vi "Live_Example_XCite.vi"() -> ()   [LabVIEW 2019]
doc: "An application to demonstrate the simultaneous control of a PCO camera and an X-Cite® light source\n\nUsage:\nSelect your required image count, data format and the camera setup before you start the program.\nOnce started, the camera class will be initialized and images will be recorded and displayed automatically\nYou can stop the images by pressing stop record.\nAfter stopped, the image at the selected index will be read out\nTo finish the program click on quit application, this will force an exit of the camera class\nYou can change your required ROI after and also during the record.\nA search for X-Cite® devices is started, and if found controls are initialized for each channel\nChannels can be switched on and off, and the intensity adjusted while the camera is acquiring images.\nWhen the recording is stopped, all the X-Cite® channels are switched off and controls are disabled.\n\n\nNote that this example will not be fail safe, i.e. doesnt react on errors, just handles them forward to the end"
uses:
  camera/Camera.lvclass
  pco.sdk/TimingControl/TimingControl.lvlib
  <vilib>/picture/picture.llb/Draw 8-Bit Pixmap.vi
  <vilib>/picture/picture.llb/Draw True-Color Pixmap.vi
  xcite/Xcite.lvclass
  <vilib>/Utility/miscctls.llb/LVOutOfRangeActionTypeDef.ctl
panel:
  in  "Channel9_On":bool caption="735 nm"
  in  "Channel9_Intensity":u32 caption="735 nm" min=5 max=100
  in  "Channel8_On":bool caption="635 nm"
  in  "Channel8_Intensity":u32 caption="635 nm" min=5 max=100
  in  "Channel7_On":bool caption="580 nm"
  in  "Channel7_Intensity":u32 caption="580 nm" min=5 max=100
  in  "Channel6_On":bool caption="555 nm"
  in  "Channel6_Intensity":u32 caption="555 nm" min=5 max=100
  in  "Channel5_On":bool caption="510 nm"
  in  "Channel5_Intensity":u32 caption="510 nm" min=5 max=100
  in  "Channel4_On":bool caption="550 nm"
  in  "Channel4_Intensity":u32 caption="550 nm" min=5 max=100
  in  "Channel3_On":bool caption="475 nm"
  in  "Channel3_Intensity":u32 caption="475 nm" min=5 max=100
  in  "Channel2_On":bool caption="430 nm"
  in  "Channel2_Intensity":u32 caption="430 nm" min=5 max=100
  in  "Channel1_On":bool caption="385 nm"
  in  "Channel1_Intensity":u32 caption="385 nm" min=5 max=100
  in  "type":u16(ring)=65535 items=["XC_120PC"=0, "XC_exacte"=1, "XC_120LED"=2, "XC_110LED"=3, "XC_mini"=4, "XC_XYLIS"=5, "XC_XR210"=6, "XC_LED1"=7, "XC_XT600"=8, "XC_XT900"=9, "Any"=65535]
  out "X-Cite® Model":u16(ring)=65535 items=["XC_120PC"=0, "XC_exacte"=1, "XC_120LED"=2, "XC_110LED"=3, "XC_mini"=4, "XC_XYLIS"=5, "XC_XR210"=6, "XC_LED1"=7, "XC_XT600"=8, "XC_XT900"=9, "Any"=65535]
  out "colormap(U8)":u32[](array[numeric])
  in  "Zoom [%]":i32(slide)=26 min=0 max=200 step=5 scale=10.0..200.0
  out "Image":picture
  out "Image(U16)":u16[][](graph)
  in  "Trigger":bool
  in  "data_format":T1(ring)=enum."Mono16"
  out "rawImage":u16[][](array[numeric])
  in  "Image Index":u32 max=9
  out "Recorded Images":u32
  in  "TriggerMode":T2(ring)
  in  "Quit":bool
  out "Error":errorcluster {"code" format="%x"}
  in  "Stop Record":bool
  out "Recording On":bool
  in  "cropY1":u64=2 min=1 max=2048 step=1
  in  "cropX1":u64=2 min=1 max=2048 step=1
  in  "cropY0":u64=1 min=1 max=2047 step=1
  in  "cropX0":u64=1 min=1 max=2047 step=1
  out "Image Height":u64
  out "Image Width":u64
  in  "dwImgCount":u32=10 caption="Required Number of Images" max=2397
  in  "Exposure Time [s]":dbl=0.010000000000000002 step=0.001
  # "This example demonstrates the image acquisition with one camera in ring buffer mode together with a live display of the latest images during record. Control of an X-Cite® light source is also possible. After recording is stopped, the images can be addressed by index.\nNote that this example will not be fail save, i.e. doesnt react on errors, just handles them forward to the end\n\nUsage:\nSelect your required image count, data format and the camera setup before you start the program.\nOnce started, the camera class will be initialized and images will be recorded and displayed automatically\nYou can stop the images by pressing stop record.\nAfter stopped, the image at the selected index will be read out\nTo finish the program click on quit application, this will force an exit of the camera class\nYou can change the cropped region during or after recording.\nA search for X-Cite® devices is started, and if found controls are initialized for each channel\nChannels can be switched on and off, and the intensity adjusted while the camera is acquiring images.\nWhen the recording is stopped, all the X-Cite® channels are switched off and controls are disabled."
  # "pco.labview"
  # "Camera Setup"
  # "X-Cite® controls"
  # "Recording Control"
  # "Parameters for image readout"
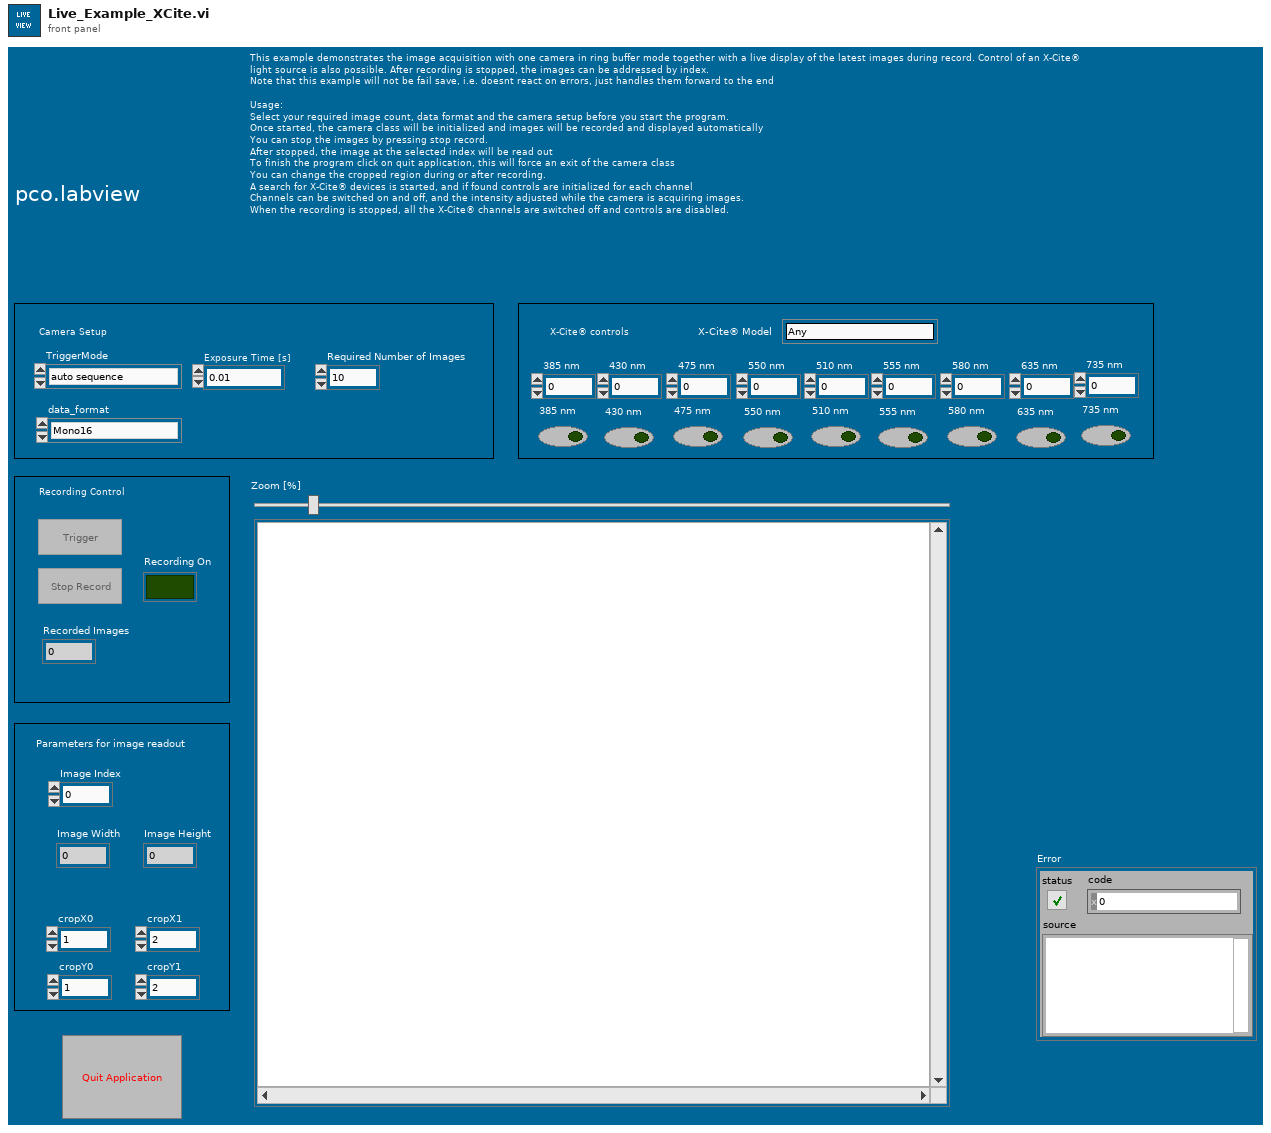
[diagram p1: front panel]
types:
  T1 = enum16{"Undefined", "Mono8", "Mono16", "BGRA8", "RGBA8", "BGRA16", "RGBA16", "CompressedMono8"}
  T2 = enum16{"auto sequence", "software trigger", "external exposure start", "external exposure control"}
  T3 = enum8{"Enabled", "Disabled", "Disabled and Grayed Out"}
  T4 = cluster{"serial":u32, "type":u16, "name":string, "wavelenghts_vec":u32[], "exclusivity_vec":u32[], "intensity_max_vec":u32[], "intensity_min_vec":u32[]}
  T5 = enum16{"sequence", "sequence non blocking", "ring buffer", "fifo", "tif", "multitif", "pcoraw", "b16", "dicom", "multidicom", "camram_ring", "camram_segment"}
  T6 = typedef "LVOutOfRangeActionTypeDef.ctl" = cluster{"Out of Range Action Minimum":u8, "Out of Range Action Maximum":u8, "Out of Range Action Increment":u8}
  T7 = cluster{"serial":u32, "type":u16, "sub_type":u16, "interface_type":u16, "bit_resolution":u16, "min_exposure_time_s":dbl, "max_exposure_time_s":dbl, "min_exposure_step_s":dbl, "min_delay_time_s":dbl, "max_delay_time_s":dbl, "min_delay_step_s":dbl, "min_width":u64, "min_height":u64, "max_width":u64, "max_height":u64, "roi_step_horz":u64, "roi_step_vert":u64, "roi_symmetric_horz":bool, "roi_symmetric_vert":bool, "has_timestamp_mode":bool, "has_timestamp_mode_ascii_only":bool, "pixelrate_vec":u32[], "conversion_factor_vec":sgl[], "has_trigger_mode_extexpctrl":bool, "has_acquire_mode":bool, "has_ext_acquire_mode":bool, "has_metadata_mode":bool, "has_ram":bool, "binning_horz_vec":u16[], "binning_vert_vec":u16[], "has_average_binning":bool, "pixel_format_vec":u32[]}
  T8 = cluster{"wSignalNum":u16, "wEnabled":u16, "wType":u16, "wPolarity":u16, "wFilterSetting":u16, "wSelected":u16, "dwParameter":u32[], "dwSignalFunctionality":u32[]}
  T9 = typedef "Camera.lvclass/binning.ctl" = cluster{"vert":u16, "horz":u16, "mode":u16}
  T10 = cluster{"exposure_time_s":dbl, "delay_time_s":dbl, "roi":cluster{"x0":u64, "y0":u64, "x1":u64, "y1":u64}, "timestamp_mode":u16, "pixelrate":u32, "conversion_factor":sgl, "trigger_mode":u16, "acquire_mode":u16, "acquire_sequence_number":u32, "metadata_mode":u16, "noisefilter_mode":u16, "pixel_format":u32, "binning":T9, "auto_exposure":cluster{"region":u16, "min_exposure_s":dbl, "max_exposure_s":dbl}}
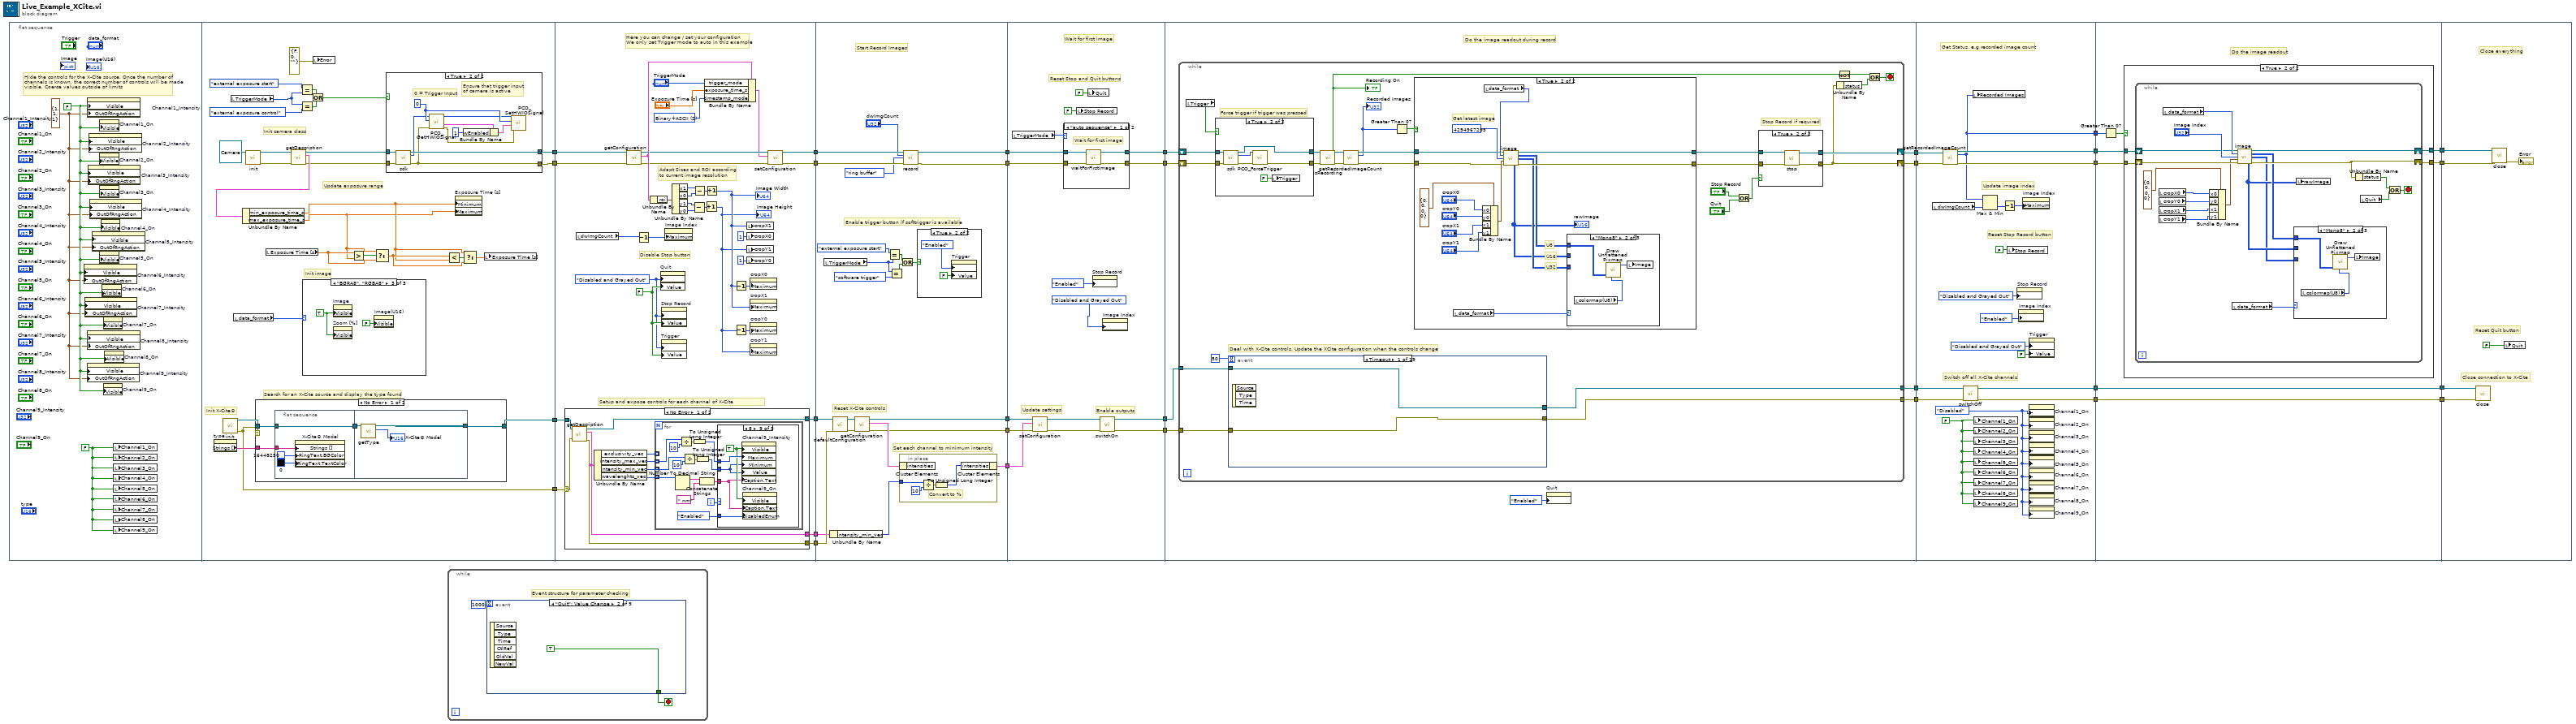
[diagram p0: block diagram]
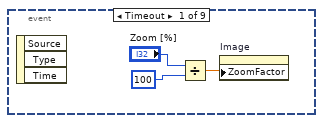
[diagram p2: hidden frame]
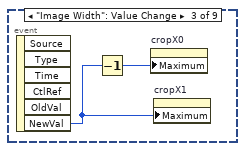
[diagram p3: hidden frame]
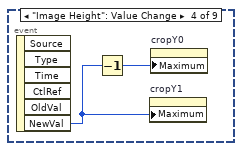
[diagram p4: hidden frame]
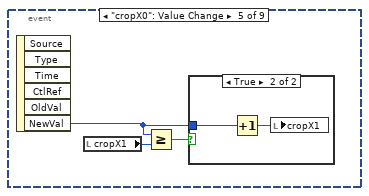
[diagram p5: hidden frame]
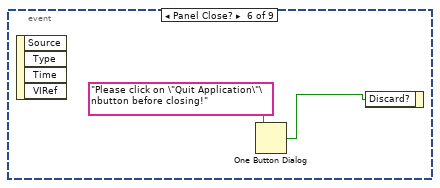
[diagram p7: hidden frame]
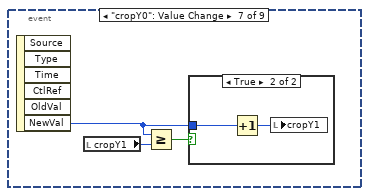
[diagram p8: hidden frame]
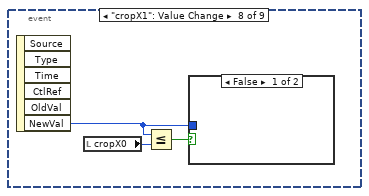
[diagram p10: hidden frame]
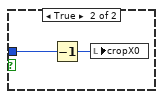
[diagram p11: hidden frame]
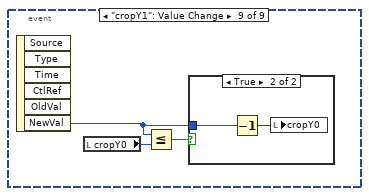
[diagram p12: hidden frame]
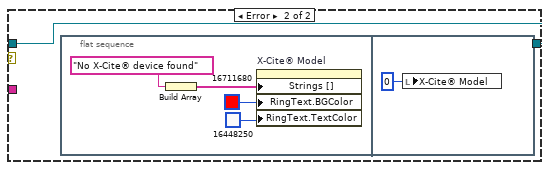
[diagram p14: hidden frame]
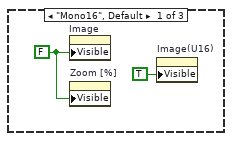
[diagram p16: hidden frame]
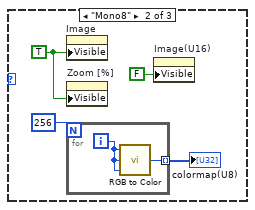
[diagram p17: hidden frame]
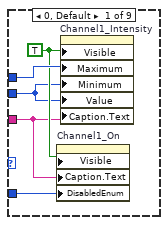
[diagram p18: hidden frame]
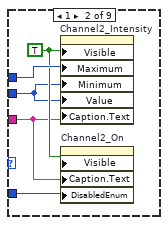
[diagram p19: hidden frame]
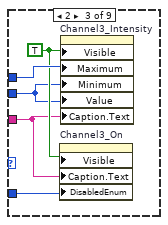
[diagram p20: hidden frame]
diagram:
  n1 = flat-sequence {
    tunnel: [w46] -> w23
    tunnel: [w39] -> w22
    tunnel: [w36] -> w16
    tunnel: [w35] -> w15
    tunnel: [w111] -> w31
    tunnel: [w115] -> w30
    tunnel: w23 -> [w110]
    tunnel: w22 -> [w109]
    tunnel: w16 -> [w105]
    tunnel: w15 -> [w106]
    tunnel: [w104] -> w14
    tunnel: [w103] -> w13
    tunnel: [w102] -> w9
    tunnel: [w217] -> w25
    tunnel: [w218] -> w24
    tunnel: w30 -> [w227]
    tunnel: w31 -> [w226]
    tunnel: w14 -> [w216]
    tunnel: w13 -> [w212]
    tunnel: w9 -> [w214]
    tunnel: [w210] -> w3
    tunnel: [w209] -> w2
    tunnel: [w207] -> w1
    tunnel: w25 -> [w245]
    tunnel: w24 -> [w246]
    tunnel: [w244] -> w29
    tunnel: [w242] -> w18
    tunnel: [w238] -> w12
    tunnel: [w239] -> w8
    tunnel: w3 -> [w236]
    tunnel: w2 -> [w240]
    tunnel: w1 -> [w234]
    tunnel: w29 -> [w264]
    tunnel: [w262] -> w28
    tunnel: [w261] -> w21
    tunnel: w18 -> [w260]
    tunnel: w12 -> [w259]
    tunnel: w8 -> [w258]
    tunnel: [w257] -> w7
    tunnel: [w256] -> w6
    tunnel: w28 -> [w609]
    tunnel: [w607] -> w27
    tunnel: w21 -> [w602]
    tunnel: [w601] -> w20
    tunnel: [w600] -> w17
    tunnel: [w599] -> w11
    tunnel: w7 -> [w598]
    tunnel: w6 -> [w597]
    tunnel: [w596] -> w5
    tunnel: w27 -> [w620]
    tunnel: [w619] -> w26
    tunnel: w20 -> [w618]
    tunnel: [w617] -> w19
    tunnel: w17 -> [w615]
    tunnel: w11 -> [w614]
    tunnel: [w614] -> w10
    tunnel: w5 -> [w613]
    tunnel: [w613] -> w4
    tunnel: w26 -> [w656]
    tunnel: w19 -> [w654]
    tunnel: w10 -> [w653]
    tunnel: w4 -> [w652]
    frame #0 {
      w32 = T6 {"Out of Range Action Minimum"=1, "Out of Range Action Maximum"=1, "Out of Range Action Increment"=1} ("Response to Value Outside Limits")
      w33 = FALSE
      w34 = FALSE
      # "Hide the controls for the X-Cite source. Once the number of channels is known, the correct number of controls will be made visible. Coerce values outside of limits"
      n2 = property on="Channel6_Intensity" class="DigNum (strict)"("Visible"=w34, "OutOfRngAction"=w32) -> ()  [unwired: 2 in, 2 out]
      n3 = property on="Channel7_Intensity" class="DigNum (strict)"("Visible"=w34, "OutOfRngAction"=w32) -> ()  [unwired: 2 in, 2 out]
      n4 = property on="Channel9_Intensity" class="DigNum (strict)"("Visible"=w34, "OutOfRngAction"=w32) -> ()  [unwired: 2 in, 2 out]
      n5 = property on="Channel1_Intensity" class="DigNum (strict)"("Visible"=w34, "OutOfRngAction"=w32) -> ()  [unwired: 2 in, 2 out]
      n6 = property on="Channel8_Intensity" class="DigNum (strict)"("Visible"=w34, "OutOfRngAction"=w32) -> ()  [unwired: 2 in, 2 out]
      n7 = property on="Channel3_Intensity" class="DigNum (strict)"("Visible"=w34, "OutOfRngAction"=w32) -> ()  [unwired: 2 in, 2 out]
      n8 = property on="Channel2_Intensity" class="DigNum (strict)"("Visible"=w34, "OutOfRngAction"=w32) -> ()  [unwired: 2 in, 2 out]
      n9 = property on="Channel4_Intensity" class="DigNum (strict)"("Visible"=w34, "OutOfRngAction"=w32) -> ()  [unwired: 2 in, 2 out]
      n10 = property on="Channel5_Intensity" class="DigNum (strict)"("Visible"=w34, "OutOfRngAction"=w32) -> ()  [unwired: 2 in, 2 out]
      n11 = property on="Channel2_On" class="Bool (strict)"("Visible"=w34) -> ()  [unwired: 2 in, 2 out]
      n12 = property on="Channel1_On" class="Bool (strict)"("Visible"=w34) -> ()  [unwired: 2 in, 2 out]
      n13 = property on="Channel3_On" class="Bool (strict)"("Visible"=w34) -> ()  [unwired: 2 in, 2 out]
      n14 = property on="Channel5_On" class="Bool (strict)"("Visible"=w34) -> ()  [unwired: 2 in, 2 out]
      n15 = property on="Channel4_On" class="Bool (strict)"("Visible"=w34) -> ()  [unwired: 2 in, 2 out]
      n16 = property on="Channel6_On" class="Bool (strict)"("Visible"=w34) -> ()  [unwired: 2 in, 2 out]
      n17 = property on="Channel7_On" class="Bool (strict)"("Visible"=w34) -> ()  [unwired: 2 in, 2 out]
      n18 = property on="Channel9_On" class="Bool (strict)"("Visible"=w34) -> ()  [unwired: 2 in, 2 out]
      n19 = property on="Channel8_On" class="Bool (strict)"("Visible"=w34) -> ()  [unwired: 2 in, 2 out]
      n20 = local write "Channel1_On"(w33) -> ()
      n21 = local write "Channel2_On"(w33) -> ()
      n22 = local write "Channel3_On"(w33) -> ()
      n23 = local write "Channel4_On"(w33) -> ()
      n24 = local write "Channel5_On"(w33) -> ()
      n25 = local write "Channel6_On"(w33) -> ()
      n26 = local write "Channel7_On"(w33) -> ()
      n27 = local write "Channel8_On"(w33) -> ()
      n28 = local write "Channel9_On"(w33) -> ()
    }
    frame #1 {
      # "Search for an X-Cite source and display the type found"
      # "Init X-Cite®"
      # "Init image"
      # "Init camera class"
      # "Update exposure range"
      n29 = property on="type" class="Ring (strict)"() -> ("Strings []"=w37:string[])  [unwired: 2 in, 2 out]
      n30 = call "init.vi"() -> ("error out"=w35:errorcluster, "Xcite out"=w38:refnum<class "Xcite.lvclass">)  [unwired: 10 in]
      n31 = local read "TriggerMode"() -> (w44:T2)
      n32 = local read "data_format"() -> (w49:T1)
      n33 = call-dynamic "init.vi"("Camera in"=refnum<class "Camera.lvclass"> refnum) -> ("Camera out"=w53:refnum<class "Camera.lvclass">, "error out"=w54:errorcluster)  [unwired: 8 in]
      n34 = case shown="No Error" w35 {
        tunnel: w38 -> [w63 w73]
        tunnel: [w64 w73] -> w36
        tunnel: w37 -> [w65 _]
        frame No Error {
          n35 = flat-sequence {
            tunnel: w65 -> [w69]
            tunnel: w63 -> [w68]
            tunnel: [w68] -> w62
            tunnel: [w72] -> w64
            tunnel: w62 -> [w70]
            frame #0 {
              n36 = property on="X-Cite® Model" class="Ring (strict)"("Strings []"=w69, "RingText.BGColor"=u32 16448250 ("Ring Text.Colors:BG Color"), "RingText.TextColor"=u32 0 ("Ring Text.Colors:FG Color")) -> ()  [unwired: 2 in, 2 out]
            }
            frame #1 {
              n37 = call "getType.vi"("Xcite in"=w70) -> ("type"=→"X-Cite® Model":u16, "Xcite out"=w72:refnum<class "Xcite.lvclass">)  [unwired: 8 in, 1 out]
            }
          }
        }
        frame Error {
          n38 = flat-sequence {
            frame #0 {
              n39 = Build Array("No X-Cite® device found") -> (w76:string[])
              n40 = property on="X-Cite® Model" class="Ring (strict)"("Strings []"=w76, "RingText.BGColor"=u32 16711680 ("Ring Text.Colors:BG Color"), "RingText.TextColor"=u32 16448250 ("Ring Text.Text Colors:Text Color")) -> ()  [unwired: 2 in, 2 out]
            }
            frame #1 {
              n41 = local write "X-Cite® Model"(0) -> ()
            }
          }
        }
      }
      n42 = local read "Exposure Time [s]"() -> (w60:dbl)
      n43 = call-dynamic "getDescription.vi"("error in (no error)"=w54, "Camera in"=w53) -> ("error out"=w48:errorcluster, "description"=w52:T7, "Camera out"=w47:refnum<class "Camera.lvclass">)  [unwired: 7 in]
      n44 = Unbundle By Name(w52) -> ("min_exposure_time_s"=w51:dbl, "max_exposure_time_s"=w50:dbl)
      n45 = Equal?(x=T2."external exposure start" ("TriggerMode"), y=w44) -> (x = y?=w42:bool)
      n46 = Equal?(x=w44, y=T2."external exposure control" ("TriggerMode")) -> (x = y?=w41:bool)
      n47 = case shown="\"BGRA8\", \"RGBA8\"" w49 {
        frame "Mono16", Default {
          w92 = FALSE ("Visible")
          n48 = property on="Image" class="Pict"("Visible"=w92) -> ()  [unwired: 2 in, 2 out]
          n49 = property on="Zoom [%]" class="Slide (strict)"("Visible"=w92) -> ()  [unwired: 2 in, 2 out]
          n50 = property on="Image(U16)" class="IntGraph (strict)"("Visible"=TRUE) -> ()  [unwired: 2 in, 2 out]
        }
        frame "Mono8" {
          w96 = TRUE ("Visible")
          n51 = property on="Image" class="Pict"("Visible"=w96) -> ()  [unwired: 2 in, 2 out]
          n52 = property on="Zoom [%]" class="Slide (strict)"("Visible"=w96) -> ()  [unwired: 2 in, 2 out]
          n53 = for {
            N: 256 -> [_]
            tunnel: [w98] -> w95 mode=indexing
            i -> [w99]
            n54 = call <vilib>:"RGB to Color.vi"("B"=w99, "G"=w99, "R"=w99) -> ("Color"=w98:u32)
          }
          "colormap(U8)" <- w95
          n55 = property on="Image(U16)" class="IntGraph (strict)"("Visible"=FALSE) -> ()  [unwired: 2 in, 2 out]
        }
        frame "BGRA8", "RGBA8" {
          w100 = TRUE ("Visible")
          n56 = property on="Image" class="Pict"("Visible"=w100) -> ()  [unwired: 2 in, 2 out]
          n57 = property on="Zoom [%]" class="Slide (strict)"("Visible"=w100) -> ()  [unwired: 2 in, 2 out]
          n58 = property on="Image(U16)" class="IntGraph (strict)"("Visible"=FALSE) -> ()  [unwired: 2 in, 2 out]
        }
      }
      n59 = Or(x=w42, y=w41) -> (x .or. y?=w40:bool)
      n60 = local write "Error"(errorcluster {"status"=FALSE, "code"=0, "source"=""} ("error IO")) -> ()
      n61 = Greater?(x=w60, y=w50) -> (0:w61:bool)
      n62 = Select(t=w50, s=w61, f=w60) -> (s? t:f=w58:dbl)
      n63 = case shown="True" w40 {
        tunnel: w48 -> [w79 w85]
        tunnel: w47 -> [w80 w84]
        tunnel: [w80 w83] -> w46
        tunnel: [w79 w81] -> w39
        frame False {
        }
        frame True {
          w89 = u16 0 ("wSignalNum")
          # "0 = Trigger Input"
          # "Ensure that trigger input\nof camera is active"
          n64 = call-dynamic "sdk.vi"("Camera in"=w84, "error in (no error)"=w85) -> ("Camera out"=w83:refnum<class "Camera.lvclass">, "sdk"=w82:u64, "error out"=w81:errorcluster)  [unwired: 11 in]
          n65 = call "PCO_GetHWIOSignal.vi"("error in (no error)"=w81, "wSignalNum"=w89, "ph"=w82) -> ("error out"=w87:errorcluster, "strSignal"=w91:T8, "ph out"=w86:u64)  [unwired: 5 in, 1 out]
          n66 = Bundle By Name(cluster=w91, "wEnabled"=u16 1) -> (w88:T8)
          n67 = call "PCO_SetHWIOSignal.vi"("error in (no error)"=w87, "strSignal"=w88, "wSignalNum"=w89, "ph"=w86) -> ()  [unwired: 5 in, 3 out]
        }
      }
      n68 = Less?(x=w58, y=w51) -> (x < y?=w59:bool)
      n69 = property on="Exposure Time [s]" class="DigNum (strict)"("Minimum"=w51, "Maximum"=w50) -> ()  [unwired: 2 in, 2 out]
      n70 = Select(t=w51, s=w59, f=w58) -> (s? t:f=w57:dbl)
      n71 = local write "Exposure Time [s]"(w57) -> ()
    }
    frame #2 {
      w121 = u16 2 items=["OFF", "Binary", "Binary+ASCII", "ASCII"] ("wTimeStampMode")
      w108 = FALSE ("Stop")
      w107 = T3."Disabled and Grayed Out" ("Disabled")
      # "Setup and expose controls for each channel of X-Cite"
      # "Disable Stop button"
      # "Adapt Sizes and ROI according\nto current image resolution"
      # "Here you can change / set your configuration\nWe only set Trigger mode to auto in this example"
      n72 = case shown="No Error" w106 {
        selector: w106 -> [w136 w203]
        tunnel: w105 -> [w143 w205]
        tunnel: [w142 w205] -> w104
        tunnel: [w137 T4 {"serial"=0, "type"=0, "name"="", "wavelenghts_vec"=[], "exclusivity_vec"=[], "intensity_max_vec"=[], "intensity_min_vec"=[]} ("XCITE_Description")] -> w103
        tunnel: [w135 w203] -> w102
        frame No Error {
          n73 = call "getDescription.vi"("error in (no error)"=w136, "Xcite in"=w143) -> ("error out"=w135:errorcluster, "description"=w137:T4, "Xcite out"=w142:refnum<class "Xcite.lvclass">)  [unwired: 7 in]
          n74 = Unbundle By Name(w137) -> ("exclusivity_vec"=w141:u32[], "intensity_max_vec"=w140:u32[], "intensity_min_vec"=w139:u32[], "wavelenghts_vec"=w138:u32[])
          n75 = for {
            tunnel: w141 -> [_] mode=indexing
            tunnel: w140 -> [w151] mode=indexing
            tunnel: w139 -> [w146] mode=indexing
            tunnel: w138 -> [w156] mode=indexing
            i -> [w157]
            n76 = Number To Decimal String(number=w156) -> (decimal integer string=w155:string)  [unwired: 1 in]
            n77 = Divide(x=w151, y=u32 10) -> (x/y=w149:dbl)
            n78 = Divide(x=w146, y=u32 10) -> (x/y=w147:dbl)
            n79 = To Unsigned Long Integer(number=w149) -> (unsigned 32bit integer=w144:u32)
            n80 = To Unsigned Long Integer(number=w147) -> (unsigned 32bit integer=w145:u32)
            n81 = Concatenate Strings(w155, " nm") -> (w153:string)
            n82 = case shown="8" w157 {
              tunnel: w153 -> [w159 w164 w169 w175 w180 w185 w189 w195 w200]
              tunnel: w144 -> [w162 w167 w172 w177 w182 w187 w192 w197 w202]
              tunnel: w145 -> [w160 w165 w170 w174 w179 w184 w190 w194 w199]
              tunnel: T3."Enabled" ("Disabled") -> [w158 w163 w168 w173 w178 w183 w188 w193 w198]
              frame 0, Default {
                w161 = TRUE ("Visible")
                n83 = property on="Channel1_On" class="Bool (strict)"("Visible"=w161, "Caption.Text"=w159, "DisabledEnum"=w158) -> ()  [unwired: 2 in, 2 out]
                n84 = property on="Channel1_Intensity" class="DigNum (strict)"("Visible"=w161, "Maximum"=w162, "Minimum"=w160, "Value"=w160, "Caption.Text"=w159) -> ()  [unwired: 2 in, 2 out]
              }
              frame 1 {
                w166 = TRUE ("Visible")
                n85 = property on="Channel2_Intensity" class="DigNum (strict)"("Visible"=w166, "Maximum"=w167, "Minimum"=w165, "Value"=w165, "Caption.Text"=w164) -> ()  [unwired: 2 in, 2 out]
                n86 = property on="Channel2_On" class="Bool (strict)"("Visible"=w166, "Caption.Text"=w164, "DisabledEnum"=w163) -> ()  [unwired: 2 in, 2 out]
              }
              frame 2 {
                w171 = TRUE ("Visible")
                n87 = property on="Channel3_On" class="Bool (strict)"("Visible"=w171, "Caption.Text"=w169, "DisabledEnum"=w168) -> ()  [unwired: 2 in, 2 out]
                n88 = property on="Channel3_Intensity" class="DigNum (strict)"("Visible"=w171, "Maximum"=w172, "Minimum"=w170, "Value"=w170, "Caption.Text"=w169) -> ()  [unwired: 2 in, 2 out]
              }
              frame 3 {
                w176 = TRUE ("Visible")
                n89 = property on="Channel4_Intensity" class="DigNum (strict)"("Visible"=w176, "Maximum"=w177, "Minimum"=w174, "Value"=w174, "Caption.Text"=w175) -> ()  [unwired: 2 in, 2 out]
                n90 = property on="Channel4_On" class="Bool (strict)"("Visible"=w176, "Caption.Text"=w175, "DisabledEnum"=w173) -> ()  [unwired: 2 in, 2 out]
              }
              frame 4 {
                w181 = TRUE ("Visible")
                n91 = property on="Channel5_Intensity" class="DigNum (strict)"("Visible"=w181, "Maximum"=w182, "Minimum"=w179, "Value"=w179, "Caption.Text"=w180) -> ()  [unwired: 2 in, 2 out]
                n92 = property on="Channel5_On" class="Bool (strict)"("Visible"=w181, "Caption.Text"=w180, "DisabledEnum"=w178) -> ()  [unwired: 2 in, 2 out]
              }
              frame 5 {
                w186 = TRUE ("Visible")
                n93 = property on="Channel6_Intensity" class="DigNum (strict)"("Visible"=w186, "Maximum"=w187, "Minimum"=w184, "Value"=w184, "Caption.Text"=w185) -> ()  [unwired: 2 in, 2 out]
                n94 = property on="Channel6_On" class="Bool (strict)"("Visible"=w186, "Caption.Text"=w185, "DisabledEnum"=w183) -> ()  [unwired: 2 in, 2 out]
              }
              frame 6 {
                w191 = TRUE ("Visible")
                n95 = property on="Channel7_Intensity" class="DigNum (strict)"("Visible"=w191, "Maximum"=w192, "Minimum"=w190, "Value"=w190, "Caption.Text"=w189) -> ()  [unwired: 2 in, 2 out]
                n96 = property on="Channel7_On" class="Bool (strict)"("Visible"=w191, "Caption.Text"=w189, "DisabledEnum"=w188) -> ()  [unwired: 2 in, 2 out]
              }
              frame 7 {
                w196 = TRUE ("Visible")
                n97 = property on="Channel8_Intensity" class="DigNum (strict)"("Visible"=w196, "Maximum"=w197, "Minimum"=w194, "Value"=w194, "Caption.Text"=w195) -> ()  [unwired: 2 in, 2 out]
                n98 = property on="Channel8_On" class="Bool (strict)"("Visible"=w196, "Caption.Text"=w195, "DisabledEnum"=w193) -> ()  [unwired: 2 in, 2 out]
              }
              frame 8 {
                w201 = TRUE ("Visible")
                n99 = property on="Channel9_Intensity" class="DigNum (strict)"("Visible"=w201, "Maximum"=w202, "Minimum"=w199, "Value"=w199, "Caption.Text"=w200) -> ()  [unwired: 2 in, 2 out]
                n100 = property on="Channel9_On" class="Bool (strict)"("Visible"=w201, "Caption.Text"=w200, "DisabledEnum"=w198) -> ()  [unwired: 2 in, 2 out]
              }
            }
          }
        }
        frame Error {
        }
      }
      n101 = local read "dwImgCount"() -> (w122:u32)
      n102 = call-dynamic "getConfiguration.vi"("error in (no error)"=w109, "Camera in"=w110) -> ("error out"=w116:errorcluster, "configuration"=w127:T10, "Camera out"=w118:refnum<class "Camera.lvclass">)  [unwired: 7 in]
      n103 = Decrement(x=w122) -> (x-1=w112:u32)
      n104 = Unbundle By Name(w127) -> ("roi"=w128:cluster{"x0":u64, "y0":u64, "x1":u64, "y1":u64})
      n105 = property on="Quit" class="Bool (strict)"("DisabledEnum"=w107, "Value"=w108) -> ()  [unwired: 2 in, 2 out]
      n106 = property on="Stop Record" class="Bool (strict)"("DisabledEnum"=w107, "Value"=w108) -> ()  [unwired: 2 in, 2 out]
      n107 = property on="Trigger" class="Bool (strict)"("DisabledEnum"=w107, "Value"=w108) -> ()  [unwired: 2 in, 2 out]
      n108 = property on="Image Index" class="DigNum (strict)"("Maximum"=w112) -> ()  [unwired: 2 in, 2 out]
      n109 = Unbundle By Name(w128) -> ("x1"=w130:u64, "x0"=w129:u64, "y1"=w132:u64, "y0"=w131:u64)
      n110 = Subtract(x=w132, y=w131) -> (x-y=w134:u64)
      n111 = Subtract(x=w130, y=w129) -> (x-y=w133:u64)
      n112 = Bundle By Name(cluster=w127, "trigger_mode"="TriggerMode", "exposure_time_s"="Exposure Time [s]", "timestamp_mode"=w121) -> (w117:T10)
      n113 = Increment(x=w134) -> (x+1=w113:u64)
      "Image Height" <- w113
      n114 = Increment(x=w133) -> (x+1=w114:u64)
      "Image Width" <- w114
      n115 = Decrement(x=w114) -> (x-1=w125:u64)
      n116 = Decrement(x=w113) -> (x-1=w126:u64)
      n117 = local write "cropX1"(w114) -> ()
      n118 = local write "cropX0"(u64 1 ("roiY0")) -> ()
      n119 = local write "cropY1"(w113) -> ()
      n120 = local write "cropY0"(u64 1 ("roiY0")) -> ()
      n121 = property on="cropX0" class="DigNum (strict)"("Maximum"=w125) -> ()  [unwired: 2 in, 2 out]
      n122 = property on="cropX1" class="DigNum (strict)"("Maximum"=w114) -> ()  [unwired: 2 in, 2 out]
      n123 = property on="cropY0" class="DigNum (strict)"("Maximum"=w126) -> ()  [unwired: 2 in, 2 out]
      n124 = property on="cropY1" class="DigNum (strict)"("Maximum"=w113) -> ()  [unwired: 2 in, 2 out]
      n125 = call-dynamic "setConfiguration.vi"("error in (no error)"=w116, "configuration"=w117, "Camera in"=w118) -> ("error out"=w115:errorcluster, "Camera out"=w111:refnum<class "Camera.lvclass">)  [unwired: 7 in]
    }
    frame #3 {
      # "Set each channel to minimum intensity"
      # "Reset X-Cite controls"
      # "Enable trigger button if softtrigger is available"
      # "Start Record Images"
      n126 = local read "TriggerMode"() -> (w223:T2)
      n127 = Unbundle By Name(w212) -> ("intensity_min_vec"=w208:u32[])
      n128 = call "defaultConfiguration.vi"("error in (no error)"=w214, "Xcite in"=w216) -> ("error out"=w213:errorcluster, "Xcite out"=w215:refnum<class "Xcite.lvclass">)  [unwired: 8 in]
      n129 = call "getConfiguration.vi"("error in (no error)"=w213, "Xcite in"=w215) -> ("error out"=w210:errorcluster, "configuration"=w211:cluster{"intensities":u32[], "on_states":u8[]}, "Xcite out"=w209:refnum<class "Xcite.lvclass">)  [unwired: 7 in]
      n130 = Equal?(x=T2."external exposure start" ("TriggerMode"), y=w223) -> (x = y?=w220:bool)
      n131 = Equal?(x=w223, y=T2."software trigger" ("TriggerMode")) -> (x = y?=w219:bool)
      n132 = in-place {
        in-place-border: w208 -> [w229]
        # "Convert to %"
        n133 = in-place-cluster #1(w211) -> ()  [unwired: 1 out]
        n134 = Divide(x=w229, y=u32 10) -> (x/y=w230:dbl[])
        n135 = To Unsigned Long Integer(number=w230) -> (unsigned 32bit integer=w228:u32[])
        n136 = in-place-cluster #1("intensities"=w228) -> (w207:cluster{"intensities":u32[], "on_states":u8[]})
      }
      n137 = Or(x=w220, y=w219) -> (x .or. y?=w221:bool)
      n138 = call-dynamic "record.vi"("Camera in"=w226, "num_images"="dwImgCount", "record_mode"=T5."ring buffer", "error in (no error)"=w227) -> ("Camera out"=w218:refnum<class "Camera.lvclass">, "error out"=w217:errorcluster)  [unwired: 10 in]
      n139 = case shown="True" w221 {
        frame False {
        }
        frame True {
          n140 = property on="Trigger" class="Bool (strict)"("DisabledEnum"=T3."Enabled" ("Disabled"), "Value"=FALSE ("Trigger")) -> ()  [unwired: 2 in, 2 out]
        }
      }
    }
    frame #4 {
      # "Enable outputs"
      # "Update settings"
      # "Wait for first image"
      # "Reset Stop and Quit buttons"
      n141 = local read "TriggerMode"() -> (w241:T2)
      n142 = call "setConfiguration.vi"("error in (no error)"=w236, "configuration"=w234, "Xcite in"=w240) -> ("error out"=w235:errorcluster, "Xcite out"=w237:refnum<class "Xcite.lvclass">)  [unwired: 7 in]
      n143 = case shown="\"auto sequence\"" w241 {
        tunnel: w246 -> [w253 w255]
        tunnel: w245 -> [w252 w254]
        tunnel: [w251 w254] -> w244
        tunnel: [w250 w255] -> w242
        frame "auto sequence" {
          # "Wait for first image"
          n144 = call-dynamic "waitForFirstImage.vi"("error in (no error)"=w252, "Camera in"=w253) -> ("error out"=w251:errorcluster, "Camera out"=w250:refnum<class "Camera.lvclass">)  [unwired: 8 in]
        }
        frame Default {
        }
      }
      n145 = local write "Stop Record"(FALSE ("Stop Record")) -> ()
      n146 = local write "Quit"(FALSE ("Stop")) -> ()
      n147 = property on="Stop Record" class="Bool (strict)"("DisabledEnum"=T3."Enabled" ("Disabled")) -> ()  [unwired: 2 in, 2 out]
      n148 = call "switchOn.vi"("error in (no error)"=w235, "Xcite in"=w237) -> ("error out"=w239:errorcluster, "Xcite out"=w238:refnum<class "Xcite.lvclass">)  [unwired: 8 in]
      n149 = property on="Image Index" class="DigNum (strict)"("DisabledEnum"=T3."Disabled and Grayed Out" ("Disabled")) -> ()  [unwired: 2 in, 2 out]
    }
    frame #5 {
      # "Do the image readout during record"
      n150 = while {
        shift-right: [w272] -> w262
        shift-left: w264 -> [w276]
        shift-right: [w273] -> w261
        shift-left: w260 -> [w277]
        tunnel: w259 -> [w268]
        tunnel: w258 -> [w267]
        tunnel: [w266] -> w257
        tunnel: [w265] -> w256
        stop <- w288 stop-if-true
        # "Deal with X-Cite controls. Update the XCite configuration when the controls change"
        # "Force trigger if trigger was pressed"
        # "Stop Record if required"
        n151 = local read "Trigger"() -> (w278:bool)
        n152 = case shown="True" w278 {
          tunnel: w277 -> [w580 w585]
          tunnel: w276 -> [w579 w584]
          tunnel: [w580 w583] -> w275
          tunnel: [w579 w582] -> w274
          frame False {
          }
          frame True {
            n153 = call-dynamic "sdk.vi"("Camera in"=w585, "error in (no error)"=w584) -> ("Camera out"=w583:refnum<class "Camera.lvclass">, "sdk"=w586:u64, "error out"=w587:errorcluster)  [unwired: 11 in]
            n154 = call "PCO_ForceTrigger.vi"("error in (no error)"=w587, "ph"=w586) -> ("error out"=w582:errorcluster)  [unwired: 6 in, 3 out]
            n155 = local write "Trigger"(FALSE ("Trigger")) -> ()
          }
        }
        n156 = event shown="[0] Timeout" {
          selector: _ -> [_ _ _ _ _ _ _ _ _ _ _ _ _ _ _ _ _ _ _]
          dyn-events: _ -> [_ _ _ _ _ _ _ _ _ _ _ _ _ _ _ _ _ _ _]
          timeout: 50 -> [_ _ _ _ _ _ _ _ _ _ _ _ _ _ _ _ _ _ _]
          tunnel: w268 -> [w292 w300 w315 w330 w345 w360 w375 w390 w405 w420 w436 w450 w464 w478 w492 w506 w520 w534 w548]
          tunnel: [w293 w299 w314 w329 w344 w359 w374 w389 w404 w419 w435 w449 w463 w477 w491 w505 w519 w533 w547] -> w265
          tunnel: w267 -> [w293 w295 w310 w325 w340 w355 w370 w385 w400 w415 w430 w444 w458 w472 w486 w500 w514 w528 w542]
          tunnel: [w292 w298 w313 w328 w343 w358 w373 w388 w403 w418 w434 w448 w462 w476 w490 w504 w518 w532 w546] -> w266
          event Timeout {
            n157 = event-data() -> ()  [unwired: 1 in, 3 out]
          }
          event "Channel1_Intensity": Value Change {
            n158 = event-data() -> ("NewVal"=w302:u32)  [unwired: 1 in, 5 out]
            n159 = call "getConfiguration.vi"("error in (no error)"=w295, "Xcite in"=w300) -> ("error out"=w294:errorcluster, "configuration"=w296:cluster{"intensities":u32[], "on_states":u8[]}, "Xcite out"=w297:refnum<class "Xcite.lvclass">)  [unwired: 7 in]
            n160 = in-place {
              in-place-border: w302 -> [w306]
              # "Convert to permille"
              n161 = in-place-cluster #2(w296) -> ("intensities"=w308:u32[])
              n162 = Replace Array Subset(array=w308, new element=w306, index=0) -> (w304:u32[])
              n163 = Multiply(x=w304, y=u32 10) -> (x*y=w303:u32[])
              n164 = in-place-cluster #2("intensities"=w303) -> (w301:cluster{"intensities":u32[], "on_states":u8[]})
            }
            n165 = call "setConfiguration.vi"("error in (no error)"=w294, "configuration"=w301, "Xcite in"=w297) -> ("error out"=w299:errorcluster, "Xcite out"=w298:refnum<class "Xcite.lvclass">)  [unwired: 7 in]
          }
          event "Channel2_Intensity": Value Change {
            n166 = event-data() -> ("NewVal"=w317:u32)  [unwired: 1 in, 5 out]
            n167 = call "getConfiguration.vi"("error in (no error)"=w310, "Xcite in"=w315) -> ("error out"=w309:errorcluster, "configuration"=w311:cluster{"intensities":u32[], "on_states":u8[]}, "Xcite out"=w312:refnum<class "Xcite.lvclass">)  [unwired: 7 in]
            n168 = in-place {
              in-place-border: w317 -> [w321]
              # "Convert to permille"
              n169 = in-place-cluster #3(w311) -> ("intensities"=w323:u32[])
              n170 = Replace Array Subset(array=w323, new element=w321, index=1) -> (w319:u32[])
              n171 = Multiply(x=w319, y=u32 10) -> (x*y=w318:u32[])
              n172 = in-place-cluster #3("intensities"=w318) -> (w316:cluster{"intensities":u32[], "on_states":u8[]})
            }
            n173 = call "setConfiguration.vi"("error in (no error)"=w309, "configuration"=w316, "Xcite in"=w312) -> ("error out"=w314:errorcluster, "Xcite out"=w313:refnum<class "Xcite.lvclass">)  [unwired: 7 in]
          }
          event "Channel3_Intensity": Value Change {
            n174 = event-data() -> ("NewVal"=w332:u32)  [unwired: 1 in, 5 out]
            n175 = call "getConfiguration.vi"("error in (no error)"=w325, "Xcite in"=w330) -> ("error out"=w324:errorcluster, "configuration"=w326:cluster{"intensities":u32[], "on_states":u8[]}, "Xcite out"=w327:refnum<class "Xcite.lvclass">)  [unwired: 7 in]
            n176 = in-place {
              in-place-border: w332 -> [w336]
              # "Convert to permille"
              n177 = in-place-cluster #4(w326) -> ("intensities"=w338:u32[])
              n178 = Replace Array Subset(array=w338, new element=w336, index=2) -> (w334:u32[])
              n179 = Multiply(x=w334, y=u32 10) -> (x*y=w333:u32[])
              n180 = in-place-cluster #4("intensities"=w333) -> (w331:cluster{"intensities":u32[], "on_states":u8[]})
            }
            n181 = call "setConfiguration.vi"("error in (no error)"=w324, "configuration"=w331, "Xcite in"=w327) -> ("error out"=w329:errorcluster, "Xcite out"=w328:refnum<class "Xcite.lvclass">)  [unwired: 7 in]
          }
          event "Channel4_Intensity": Value Change {
            n182 = event-data() -> ("NewVal"=w347:u32)  [unwired: 1 in, 5 out]
            n183 = call "getConfiguration.vi"("error in (no error)"=w340, "Xcite in"=w345) -> ("error out"=w339:errorcluster, "configuration"=w341:cluster{"intensities":u32[], "on_states":u8[]}, "Xcite out"=w342:refnum<class "Xcite.lvclass">)  [unwired: 7 in]
            n184 = in-place {
              in-place-border: w347 -> [w351]
              # "Convert to permille"
              n185 = in-place-cluster #5(w341) -> ("intensities"=w353:u32[])
              n186 = Replace Array Subset(array=w353, new element=w351, index=3) -> (w349:u32[])
              n187 = Multiply(x=w349, y=u32 10) -> (x*y=w348:u32[])
              n188 = in-place-cluster #5("intensities"=w348) -> (w346:cluster{"intensities":u32[], "on_states":u8[]})
            }
            n189 = call "setConfiguration.vi"("error in (no error)"=w339, "configuration"=w346, "Xcite in"=w342) -> ("error out"=w344:errorcluster, "Xcite out"=w343:refnum<class "Xcite.lvclass">)  [unwired: 7 in]
          }
          event "Channel5_Intensity": Value Change {
            n190 = event-data() -> ("NewVal"=w362:u32)  [unwired: 1 in, 5 out]
            n191 = call "getConfiguration.vi"("error in (no error)"=w355, "Xcite in"=w360) -> ("error out"=w354:errorcluster, "configuration"=w356:cluster{"intensities":u32[], "on_states":u8[]}, "Xcite out"=w357:refnum<class "Xcite.lvclass">)  [unwired: 7 in]
            n192 = in-place {
              in-place-border: w362 -> [w366]
              # "Convert to permille"
              n193 = in-place-cluster #6(w356) -> ("intensities"=w368:u32[])
              n194 = Replace Array Subset(array=w368, new element=w366, index=4) -> (w364:u32[])
              n195 = Multiply(x=w364, y=u32 10) -> (x*y=w363:u32[])
              n196 = in-place-cluster #6("intensities"=w363) -> (w361:cluster{"intensities":u32[], "on_states":u8[]})
            }
            n197 = call "setConfiguration.vi"("error in (no error)"=w354, "configuration"=w361, "Xcite in"=w357) -> ("error out"=w359:errorcluster, "Xcite out"=w358:refnum<class "Xcite.lvclass">)  [unwired: 7 in]
          }
          event "Channel6_Intensity": Value Change {
            n198 = event-data() -> ("NewVal"=w377:u32)  [unwired: 1 in, 5 out]
            n199 = call "getConfiguration.vi"("error in (no error)"=w370, "Xcite in"=w375) -> ("error out"=w369:errorcluster, "configuration"=w371:cluster{"intensities":u32[], "on_states":u8[]}, "Xcite out"=w372:refnum<class "Xcite.lvclass">)  [unwired: 7 in]
            n200 = in-place {
              in-place-border: w377 -> [w381]
              # "Convert to permille"
              n201 = in-place-cluster #7(w371) -> ("intensities"=w383:u32[])
              n202 = Replace Array Subset(array=w383, new element=w381, index=5) -> (w379:u32[])
              n203 = Multiply(x=w379, y=u32 10) -> (x*y=w378:u32[])
              n204 = in-place-cluster #7("intensities"=w378) -> (w376:cluster{"intensities":u32[], "on_states":u8[]})
            }
            n205 = call "setConfiguration.vi"("error in (no error)"=w369, "configuration"=w376, "Xcite in"=w372) -> ("error out"=w374:errorcluster, "Xcite out"=w373:refnum<class "Xcite.lvclass">)  [unwired: 7 in]
          }
          event "Channel7_Intensity": Value Change {
            n206 = event-data() -> ("NewVal"=w392:u32)  [unwired: 1 in, 5 out]
            n207 = call "getConfiguration.vi"("error in (no error)"=w385, "Xcite in"=w390) -> ("error out"=w384:errorcluster, "configuration"=w386:cluster{"intensities":u32[], "on_states":u8[]}, "Xcite out"=w387:refnum<class "Xcite.lvclass">)  [unwired: 7 in]
            n208 = in-place {
              in-place-border: w392 -> [w396]
              # "Convert to permille"
              n209 = in-place-cluster #8(w386) -> ("intensities"=w398:u32[])
              n210 = Replace Array Subset(array=w398, new element=w396, index=6) -> (w394:u32[])
              n211 = Multiply(x=w394, y=u32 10) -> (x*y=w393:u32[])
              n212 = in-place-cluster #8("intensities"=w393) -> (w391:cluster{"intensities":u32[], "on_states":u8[]})
            }
            n213 = call "setConfiguration.vi"("error in (no error)"=w384, "configuration"=w391, "Xcite in"=w387) -> ("error out"=w389:errorcluster, "Xcite out"=w388:refnum<class "Xcite.lvclass">)  [unwired: 7 in]
          }
          event "Channel8_Intensity": Value Change {
            n214 = event-data() -> ("NewVal"=w407:u32)  [unwired: 1 in, 5 out]
            n215 = call "getConfiguration.vi"("error in (no error)"=w400, "Xcite in"=w405) -> ("error out"=w399:errorcluster, "configuration"=w401:cluster{"intensities":u32[], "on_states":u8[]}, "Xcite out"=w402:refnum<class "Xcite.lvclass">)  [unwired: 7 in]
            n216 = in-place {
              in-place-border: w407 -> [w411]
              # "Convert to permille"
              n217 = in-place-cluster #9(w401) -> ("intensities"=w413:u32[])
              n218 = Replace Array Subset(array=w413, new element=w411, index=7) -> (w409:u32[])
              n219 = Multiply(x=w409, y=u32 10) -> (x*y=w408:u32[])
              n220 = in-place-cluster #9("intensities"=w408) -> (w406:cluster{"intensities":u32[], "on_states":u8[]})
            }
            n221 = call "setConfiguration.vi"("error in (no error)"=w399, "configuration"=w406, "Xcite in"=w402) -> ("error out"=w404:errorcluster, "Xcite out"=w403:refnum<class "Xcite.lvclass">)  [unwired: 7 in]
          }
          event "Channel9_Intensity": Value Change {
            n222 = event-data() -> ("NewVal"=w422:u32)  [unwired: 1 in, 5 out]
            n223 = call "getConfiguration.vi"("error in (no error)"=w415, "Xcite in"=w420) -> ("error out"=w414:errorcluster, "configuration"=w416:cluster{"intensities":u32[], "on_states":u8[]}, "Xcite out"=w417:refnum<class "Xcite.lvclass">)  [unwired: 7 in]
            n224 = in-place {
              in-place-border: w422 -> [w426]
              # "Convert to permille"
              n225 = in-place-cluster #10(w416) -> ("intensities"=w428:u32[])
              n226 = Replace Array Subset(array=w428, new element=w426, index=8) -> (w424:u32[])
              n227 = Multiply(x=w424, y=u32 10) -> (x*y=w423:u32[])
              n228 = in-place-cluster #10("intensities"=w423) -> (w421:cluster{"intensities":u32[], "on_states":u8[]})
            }
            n229 = call "setConfiguration.vi"("error in (no error)"=w414, "configuration"=w421, "Xcite in"=w417) -> ("error out"=w419:errorcluster, "Xcite out"=w418:refnum<class "Xcite.lvclass">)  [unwired: 7 in]
          }
          event "Channel1_On": Value Change {
            n230 = event-data() -> ("NewVal"=w438:bool)  [unwired: 1 in, 5 out]
            n231 = call "getConfiguration.vi"("error in (no error)"=w430, "Xcite in"=w436) -> ("error out"=w429:errorcluster, "configuration"=w432:cluster{"intensities":u32[], "on_states":u8[]}, "Xcite out"=w433:refnum<class "Xcite.lvclass">)  [unwired: 7 in]
            n232 = Boolean To (0,1)(Boolean=w438) -> (0, 1=w431:i16)
            n233 = in-place {
              in-place-border: w431 -> [w439]
              n234 = in-place-cluster #11(w432) -> ("on_states"=w442:u8[])
              n235 = Replace Array Subset(array=w442, new element=w439, index=0) -> (w441:u8[])
              n236 = in-place-cluster #11("on_states"=w441) -> (w437:cluster{"intensities":u32[], "on_states":u8[]})
            }
            n237 = call "setConfiguration.vi"("error in (no error)"=w429, "configuration"=w437, "Xcite in"=w433) -> ("error out"=w435:errorcluster, "Xcite out"=w434:refnum<class "Xcite.lvclass">)  [unwired: 7 in]
          }
          event "Channel2_On": Value Change {
            n238 = event-data() -> ("NewVal"=w452:bool)  [unwired: 1 in, 5 out]
            n239 = Boolean To (0,1)(Boolean=w452) -> (0, 1=w445:i16)
            n240 = call "getConfiguration.vi"("error in (no error)"=w444, "Xcite in"=w450) -> ("error out"=w443:errorcluster, "configuration"=w446:cluster{"intensities":u32[], "on_states":u8[]}, "Xcite out"=w447:refnum<class "Xcite.lvclass">)  [unwired: 7 in]
            n241 = in-place {
              in-place-border: w445 -> [w453]
              n242 = in-place-cluster #12(w446) -> ("on_states"=w456:u8[])
              n243 = Replace Array Subset(array=w456, new element=w453, index=1) -> (w455:u8[])
              n244 = in-place-cluster #12("on_states"=w455) -> (w451:cluster{"intensities":u32[], "on_states":u8[]})
            }
            n245 = call "setConfiguration.vi"("error in (no error)"=w443, "configuration"=w451, "Xcite in"=w447) -> ("error out"=w449:errorcluster, "Xcite out"=w448:refnum<class "Xcite.lvclass">)  [unwired: 7 in]
          }
          event "Channel3_On": Value Change {
            n246 = event-data() -> ("NewVal"=w466:bool)  [unwired: 1 in, 5 out]
            n247 = call "getConfiguration.vi"("error in (no error)"=w458, "Xcite in"=w464) -> ("error out"=w457:errorcluster, "configuration"=w460:cluster{"intensities":u32[], "on_states":u8[]}, "Xcite out"=w461:refnum<class "Xcite.lvclass">)  [unwired: 7 in]
            n248 = Boolean To (0,1)(Boolean=w466) -> (0, 1=w459:i16)
            n249 = in-place {
              in-place-border: w459 -> [w467]
              n250 = in-place-cluster #13(w460) -> ("on_states"=w470:u8[])
              n251 = Replace Array Subset(array=w470, new element=w467, index=2) -> (w469:u8[])
              n252 = in-place-cluster #13("on_states"=w469) -> (w465:cluster{"intensities":u32[], "on_states":u8[]})
            }
            n253 = call "setConfiguration.vi"("error in (no error)"=w457, "configuration"=w465, "Xcite in"=w461) -> ("error out"=w463:errorcluster, "Xcite out"=w462:refnum<class "Xcite.lvclass">)  [unwired: 7 in]
          }
          event "Channel4_On": Value Change {
            n254 = event-data() -> ("NewVal"=w480:bool)  [unwired: 1 in, 5 out]
            n255 = call "getConfiguration.vi"("error in (no error)"=w472, "Xcite in"=w478) -> ("error out"=w471:errorcluster, "configuration"=w474:cluster{"intensities":u32[], "on_states":u8[]}, "Xcite out"=w475:refnum<class "Xcite.lvclass">)  [unwired: 7 in]
            n256 = Boolean To (0,1)(Boolean=w480) -> (0, 1=w473:i16)
            n257 = in-place {
              in-place-border: w473 -> [w481]
              n258 = in-place-cluster #14(w474) -> ("on_states"=w484:u8[])
              n259 = Replace Array Subset(array=w484, new element=w481, index=3) -> (w483:u8[])
              n260 = in-place-cluster #14("on_states"=w483) -> (w479:cluster{"intensities":u32[], "on_states":u8[]})
            }
            n261 = call "setConfiguration.vi"("error in (no error)"=w471, "configuration"=w479, "Xcite in"=w475) -> ("error out"=w477:errorcluster, "Xcite out"=w476:refnum<class "Xcite.lvclass">)  [unwired: 7 in]
          }
          event "Channel5_On": Value Change {
            n262 = event-data() -> ("NewVal"=w494:bool)  [unwired: 1 in, 5 out]
            n263 = call "getConfiguration.vi"("error in (no error)"=w486, "Xcite in"=w492) -> ("error out"=w485:errorcluster, "configuration"=w488:cluster{"intensities":u32[], "on_states":u8[]}, "Xcite out"=w489:refnum<class "Xcite.lvclass">)  [unwired: 7 in]
            n264 = Boolean To (0,1)(Boolean=w494) -> (0, 1=w487:i16)
            n265 = in-place {
              in-place-border: w487 -> [w495]
              n266 = in-place-cluster #15(w488) -> ("on_states"=w498:u8[])
              n267 = Replace Array Subset(array=w498, new element=w495, index=4) -> (w497:u8[])
              n268 = in-place-cluster #15("on_states"=w497) -> (w493:cluster{"intensities":u32[], "on_states":u8[]})
            }
            n269 = call "setConfiguration.vi"("error in (no error)"=w485, "configuration"=w493, "Xcite in"=w489) -> ("error out"=w491:errorcluster, "Xcite out"=w490:refnum<class "Xcite.lvclass">)  [unwired: 7 in]
          }
          event "Channel6_On": Value Change {
            n270 = event-data() -> ("NewVal"=w508:bool)  [unwired: 1 in, 5 out]
            n271 = call "getConfiguration.vi"("error in (no error)"=w500, "Xcite in"=w506) -> ("error out"=w499:errorcluster, "configuration"=w502:cluster{"intensities":u32[], "on_states":u8[]}, "Xcite out"=w503:refnum<class "Xcite.lvclass">)  [unwired: 7 in]
            n272 = Boolean To (0,1)(Boolean=w508) -> (0, 1=w501:i16)
            n273 = in-place {
              in-place-border: w501 -> [w509]
              n274 = in-place-cluster #16(w502) -> ("on_states"=w512:u8[])
              n275 = Replace Array Subset(array=w512, new element=w509, index=5) -> (w511:u8[])
              n276 = in-place-cluster #16("on_states"=w511) -> (w507:cluster{"intensities":u32[], "on_states":u8[]})
            }
            n277 = call "setConfiguration.vi"("error in (no error)"=w499, "configuration"=w507, "Xcite in"=w503) -> ("error out"=w505:errorcluster, "Xcite out"=w504:refnum<class "Xcite.lvclass">)  [unwired: 7 in]
          }
          event "Channel7_On": Value Change {
            n278 = event-data() -> ("NewVal"=w522:bool)  [unwired: 1 in, 5 out]
            n279 = call "getConfiguration.vi"("error in (no error)"=w514, "Xcite in"=w520) -> ("error out"=w513:errorcluster, "configuration"=w516:cluster{"intensities":u32[], "on_states":u8[]}, "Xcite out"=w517:refnum<class "Xcite.lvclass">)  [unwired: 7 in]
            n280 = Boolean To (0,1)(Boolean=w522) -> (0, 1=w515:i16)
            n281 = in-place {
              in-place-border: w515 -> [w523]
              n282 = in-place-cluster #17(w516) -> ("on_states"=w526:u8[])
              n283 = Replace Array Subset(array=w526, new element=w523, index=6) -> (w525:u8[])
              n284 = in-place-cluster #17("on_states"=w525) -> (w521:cluster{"intensities":u32[], "on_states":u8[]})
            }
            n285 = call "setConfiguration.vi"("error in (no error)"=w513, "configuration"=w521, "Xcite in"=w517) -> ("error out"=w519:errorcluster, "Xcite out"=w518:refnum<class "Xcite.lvclass">)  [unwired: 7 in]
          }
          event "Channel8_On": Value Change {
            n286 = event-data() -> ("NewVal"=w536:bool)  [unwired: 1 in, 5 out]
            n287 = call "getConfiguration.vi"("error in (no error)"=w528, "Xcite in"=w534) -> ("error out"=w527:errorcluster, "configuration"=w530:cluster{"intensities":u32[], "on_states":u8[]}, "Xcite out"=w531:refnum<class "Xcite.lvclass">)  [unwired: 7 in]
            n288 = Boolean To (0,1)(Boolean=w536) -> (0, 1=w529:i16)
            n289 = in-place {
              in-place-border: w529 -> [w537]
              n290 = in-place-cluster #18(w530) -> ("on_states"=w540:u8[])
              n291 = Replace Array Subset(array=w540, new element=w537, index=7) -> (w539:u8[])
              n292 = in-place-cluster #18("on_states"=w539) -> (w535:cluster{"intensities":u32[], "on_states":u8[]})
            }
            n293 = call "setConfiguration.vi"("error in (no error)"=w527, "configuration"=w535, "Xcite in"=w531) -> ("error out"=w533:errorcluster, "Xcite out"=w532:refnum<class "Xcite.lvclass">)  [unwired: 7 in]
          }
          event "Channel9_On": Value Change {
            n294 = event-data() -> ("NewVal"=w550:bool)  [unwired: 1 in, 5 out]
            n295 = call "getConfiguration.vi"("error in (no error)"=w542, "Xcite in"=w548) -> ("error out"=w541:errorcluster, "configuration"=w544:cluster{"intensities":u32[], "on_states":u8[]}, "Xcite out"=w545:refnum<class "Xcite.lvclass">)  [unwired: 7 in]
            n296 = Boolean To (0,1)(Boolean=w550) -> (0, 1=w543:i16)
            n297 = in-place {
              in-place-border: w543 -> [w551]
              n298 = in-place-cluster #19(w544) -> ("on_states"=w554:u8[])
              n299 = Replace Array Subset(array=w554, new element=w551, index=8) -> (w553:u8[])
              n300 = in-place-cluster #19("on_states"=w553) -> (w549:cluster{"intensities":u32[], "on_states":u8[]})
            }
            n301 = call "setConfiguration.vi"("error in (no error)"=w541, "configuration"=w549, "Xcite in"=w545) -> ("error out"=w547:errorcluster, "Xcite out"=w546:refnum<class "Xcite.lvclass">)  [unwired: 7 in]
          }
        }
        n302 = call-dynamic "isRecording.vi"("Camera in"=w275, "error in (no error)"=w274) -> ("Camera out"=w283:refnum<class "Camera.lvclass">, "recording"=w286:bool, "error out"=w282:errorcluster)  [unwired: 11 in]
        "Recording On" <- w286
        n303 = call-dynamic "getRecordedImageCount.vi"("Camera in"=w283, "error in (no error)"=w282) -> ("Camera out"=w280:refnum<class "Camera.lvclass">, "recorded_image_count"=w270:u32, "error out"=w281:errorcluster)  [unwired: 11 in]
        "Recorded Images" <- w270
        n304 = Greater Than 0?(x=w270) -> (x > 0?=w271:bool)
        n305 = case shown="True" w271 {
          tunnel: [w555 w567] -> w284
          tunnel: w281 -> [w555 w564]
          tunnel: w280 -> [w556 w558]
          tunnel: [w556 w557] -> w279
          frame False {
          }
          frame True {
            # "U32"
            # "U8"
            # "U16"
            # "Get latest image"
            n306 = local read "data_format"() -> (w559:T1)
            n307 = Bundle By Name(cluster=cluster{"x0":u64, "y0":u64, "x1":u64, "y1":u64} {"x0"=0, "y0"=0, "x1"=0, "y1"=0} ("roi"), "x0"="cropX0", "y0"="cropY0", "x1"="cropX1", "y1"="cropY1") -> (w568:cluster{"x0":u64, "y0":u64, "x1":u64, "y1":u64})
            n308 = local read "data_format"() -> (w563:T1)
            n309 = call-dynamic "image.vi"("Camera in"=w558, "data_format"=w563, "image_index"=u32 4294967295 ("dwImgIdx"), "crop"=w568, "error in (no error)"=w564) -> ("Camera out"=w557:refnum<class "Camera.lvclass">, "image (U8)"=w561:u8[][], "image (U32)"=w562:u32[][], "raw_image (U16)"=w560:u16[][], "error out"=w567:errorcluster)  [unwired: 2 in, 4 out]
            "rawImage" <- w560
            n310 = case shown="\"Mono8\"" w559 {
              tunnel: w562 -> [_ _ w578]
              tunnel: w561 -> [_ w576 _]
              tunnel: w560 -> [w573 _ _]
              frame "Mono16", Default {
                n311 = local write "Image(U16)"(w573) -> ()
              }
              frame "Mono8" {
                n312 = local read "colormap(U8)"() -> (w575:u32[])
                n313 = call-poly <vilib>:"Draw Unflattened Pixmap.vi"("data"=w576, "color table"=w575) -> ("new picture"=w574:picture)  [unwired: 7 in]
                n314 = local write "Image"(w574) -> ()
              }
              frame "BGRA8", "RGBA8" {
                n315 = call-poly <vilib>:"Draw Unflattened Pixmap.vi"("data (RGB format)"=w578) -> ("new picture"=w577:picture)  [unwired: 8 in]
                n316 = local write "Image"(w577) -> ()
              }
            }
          }
        }
        n317 = Or(x="Stop Record", y="Quit") -> (x .or. y?=w289:bool)
        n318 = case shown="True" w289 {
          tunnel: w284 -> [w589 w590]
          tunnel: [w588 w592] -> w273
          tunnel: [w589 w593] -> w272
          tunnel: w279 -> [w588 w591]
          frame False {
          }
          frame True {
            n319 = call-dynamic "stop.vi"("error in (no error)"=w590, "Camera in"=w591) -> ("error out"=w593:errorcluster, "Camera out"=w592:refnum<class "Camera.lvclass">)  [unwired: 8 in]
          }
        }
        n320 = Unbundle By Name(w272) -> ("status"=w287:bool)
        n321 = Not(x=w286) -> (.not. x?=w285:bool)
        n322 = Or(x=w285, y=w287) -> (x .or. y?=w288:bool)
      }
      n323 = property on="Quit" class="Bool (strict)"("DisabledEnum"=T3."Enabled" ("Disabled")) -> ()  [unwired: 2 in, 2 out]
    }
    frame #6 {
      w594 = T3."Disabled" ("Disabled")
      w595 = FALSE
      # "Switch off all X-Cite channels"
      # "Update image index"
      # "Reset Stop Record button"
      # "Get Status, e.g recorded image count"
      n324 = local read "dwImgCount"() -> (w608:u32)
      n325 = call-dynamic "getRecordedImageCount.vi"("Camera in"=w602, "error in (no error)"=w609) -> ("Camera out"=w601:refnum<class "Camera.lvclass">, "recorded_image_count"=w600:u32, "error out"=w607:errorcluster)  [unwired: 11 in]
      n326 = call "switchOff.vi"("error in (no error)"=w597, "Xcite in"=w598) -> ("error out"=w596:errorcluster, "Xcite out"=w599:refnum<class "Xcite.lvclass">)  [unwired: 8 in]
      n327 = local write "Recorded Images"(w600) -> ()
      n328 = local write "Channel1_On"(w595) -> ()
      n329 = local write "Channel2_On"(w595) -> ()
      n330 = local write "Channel3_On"(w595) -> ()
      n331 = local write "Channel4_On"(w595) -> ()
      n332 = local write "Channel5_On"(w595) -> ()
      n333 = local write "Channel6_On"(w595) -> ()
      n334 = local write "Channel7_On"(w595) -> ()
      n335 = local write "Channel8_On"(w595) -> ()
      n336 = local write "Channel9_On"(w595) -> ()
      n337 = Max & Min(x=w600, y=w608) -> (min(x,y)=w610:u32)  [unwired: 1 out]
      n338 = Decrement(x=w610) -> (x-1=w605:u32)
      n339 = local write "Stop Record"(FALSE ("Stop Record")) -> ()
      n340 = property on="Stop Record" class="Bool (strict)"("DisabledEnum"=T3."Disabled and Grayed Out" ("Disabled")) -> ()  [unwired: 2 in, 2 out]
      n341 = property on="Image Index" class="DigNum (strict)"("DisabledEnum"=T3."Enabled" ("Disabled")) -> ()  [unwired: 2 in, 2 out]
      n342 = property on="Image Index" class="DigNum (strict)"("Maximum"=w605) -> ()  [unwired: 2 in, 2 out]
      n343 = property on="Trigger" class="Bool (strict)"("DisabledEnum"=T3."Disabled and Grayed Out" ("Disabled"), "Value"=FALSE ("Trigger")) -> ()  [unwired: 2 in, 2 out]
      n344 = property on="Channel1_On" class="Bool (strict)"("DisabledEnum"=w594) -> ()  [unwired: 2 in, 2 out]
      n345 = property on="Channel2_On" class="Bool (strict)"("DisabledEnum"=w594) -> ()  [unwired: 2 in, 2 out]
      n346 = property on="Channel3_On" class="Bool (strict)"("DisabledEnum"=w594) -> ()  [unwired: 2 in, 2 out]
      n347 = property on="Channel4_On" class="Bool (strict)"("DisabledEnum"=w594) -> ()  [unwired: 2 in, 2 out]
      n348 = property on="Channel5_On" class="Bool (strict)"("DisabledEnum"=w594) -> ()  [unwired: 2 in, 2 out]
      n349 = property on="Channel6_On" class="Bool (strict)"("DisabledEnum"=w594) -> ()  [unwired: 2 in, 2 out]
      n350 = property on="Channel7_On" class="Bool (strict)"("DisabledEnum"=w594) -> ()  [unwired: 2 in, 2 out]
      n351 = property on="Channel8_On" class="Bool (strict)"("DisabledEnum"=w594) -> ()  [unwired: 2 in, 2 out]
      n352 = property on="Channel9_On" class="Bool (strict)"("DisabledEnum"=w594) -> ()  [unwired: 2 in, 2 out]
    }
    frame #7 {
      # "Do the image readout"
      n353 = Greater Than 0?(x=w615) -> (x > 0?=w616:bool)
      n354 = case shown="True" w616 {
        tunnel: w620 -> [w621 w626]
        tunnel: [w621 w625] -> w619
        tunnel: w618 -> [w622 w624]
        tunnel: [w622 w623] -> w617
        frame False {
        }
        frame True {
          n355 = while {
            shift-right: [w637] -> w625
            shift-left: w626 -> [w645]
            shift-right: [w631] -> w623
            shift-left: w624 -> [w632]
            stop <- w639 stop-if-true
            n356 = local read "cropX0"() -> (w635:u64)
            n357 = local read "cropY0"() -> (w636:u64)
            n358 = local read "cropX1"() -> (w643:u64)
            n359 = local read "cropY1"() -> (w642:u64)
            n360 = local read "data_format"() -> (w633:T1)
            n361 = Bundle By Name(cluster=cluster{"x0":u64, "y0":u64, "x1":u64, "y1":u64} {"x0"=0, "y0"=0, "x1"=0, "y1"=0} ("roi"), "x0"=w635, "y0"=w636, "x1"=w643, "y1"=w642) -> (w644:cluster{"x0":u64, "y0":u64, "x1":u64, "y1":u64})
            n362 = local read "data_format"() -> (w630:T1)
            n363 = call-dynamic "image.vi"("Camera in"=w632, "data_format"=w633, "image_index"="Image Index", "crop"=w644, "error in (no error)"=w645) -> ("Camera out"=w631:refnum<class "Camera.lvclass">, "image (U8)"=w629:u8[][], "image (U32)"=w627:u32[][], "raw_image (U16)"=w628:u16[][], "error out"=w637:errorcluster)  [unwired: 2 in, 4 out]
            n364 = case shown="\"Mono8\"" w630 {
              tunnel: w627 -> [_ _ w651]
              tunnel: w629 -> [_ w649 _]
              tunnel: w628 -> [w646 _ _]
              frame "Mono16", Default {
                n365 = local write "Image(U16)"(w646) -> ()
              }
              frame "Mono8" {
                n366 = local read "colormap(U8)"() -> (w648:u32[])
                n367 = call-poly <vilib>:"Draw Unflattened Pixmap.vi"("data"=w649, "color table"=w648) -> ("new picture"=w647:picture)  [unwired: 7 in]
                n368 = local write "Image"(w647) -> ()
              }
              frame "BGRA8", "RGBA8" {
                n369 = call-poly <vilib>:"Draw Unflattened Pixmap.vi"("data (RGB format)"=w651) -> ("new picture"=w650:picture)  [unwired: 8 in]
                n370 = local write "Image"(w650) -> ()
              }
            }
            n371 = local write "rawImage"(w628) -> ()
            n372 = Unbundle By Name(w637) -> ("status"=w640:bool)
            n373 = local read "Quit"() -> (w641:bool)
            n374 = Or(x=w640, y=w641) -> (x .or. y?=w639:bool)
          }
        }
      }
    }
    frame #8 {
      # "Close connection to X-Cite"
      # "Close everything"
      # "Reset Quit button"
      n375 = call "close.vi"("error in (no error)"=w652, "Xcite in"=w653) -> ()  [unwired: 9 in, 1 out]
      n376 = call-dynamic "close.vi"("error in (no error)"=w656, "Camera in"=w654) -> ("error out"=→"Error":errorcluster)  [unwired: 9 in]
      n377 = local write "Quit"(FALSE ("Stop Record")) -> ()
    }
  }
  n378 = while {
    stop <- w658 stop-if-true
    # "Event structure for parameter checking"
    n379 = event shown="[1] \"Quit\": Value Change" {
      selector: _ -> [_ _ _ _ _ _ _ _ _]
      dyn-events: _ -> [_ _ _ _ _ _ _ _ _]
      timeout: 1000 -> [_ _ _ _ _ _ _ _ _]
      tunnel: [_ TRUE _ _ _ _ _ _ _] -> w658
      event Timeout {
        n380 = event-data() -> ()  [unwired: 1 in, 3 out]
        n381 = Divide(x="Zoom [%]", y=100 ("Zoom [%]")) -> (x/y=w661:dbl)
        n382 = property on="Image" class="Pict"("ZoomFactor"=w661) -> ()  [unwired: 2 in, 2 out]
      }
      event "Quit": Value Change {
        n383 = event-data() -> ()  [unwired: 1 in, 6 out]
      }
      event "Image Width": Value Change {
        n384 = event-data() -> ("NewVal"=w664:u64)  [unwired: 1 in, 5 out]
        n385 = Decrement(x=w664) -> (x-1=w665:u64)
        n386 = property on="cropX0" class="DigNum (strict)"("Maximum"=w665) -> ()  [unwired: 2 in, 2 out]
        n387 = property on="cropX1" class="DigNum (strict)"("Maximum"=w664) -> ()  [unwired: 2 in, 2 out]
      }
      event "Image Height": Value Change {
        n388 = event-data() -> ("NewVal"=w666:u64)  [unwired: 1 in, 5 out]
        n389 = Decrement(x=w666) -> (x-1=w667:u64)
        n390 = property on="cropY1" class="DigNum (strict)"("Maximum"=w666) -> ()  [unwired: 2 in, 2 out]
        n391 = property on="cropY0" class="DigNum (strict)"("Maximum"=w667) -> ()  [unwired: 2 in, 2 out]
      }
      event "cropX0": Value Change {
        n392 = event-data() -> ("NewVal"=w668:u64)  [unwired: 1 in, 5 out]
        n393 = local read "cropX1"() -> (w670:u64)
        n394 = Greater Or Equal?(x=w668, y=w670) -> (x >= y?=w669:bool)
        n395 = case shown="True" w669 {
          tunnel: w668 -> [_ w672]
          frame False {
          }
          frame True {
            n396 = Increment(x=w672) -> (x+1=w671:u64)
            n397 = local write "cropX1"(w671) -> ()
          }
        }
      }
      event Panel Close? {
        n398 = event-data() -> ()  [unwired: 1 in, 4 out]
        n399 = One Button Dialog(message="Please click on \"Quit Application\"\nbutton before closing!") -> (true=w673:bool)  [unwired: 1 in]
        n400 = event-data("Discard?"=w673) -> ()  [unwired: 1 in, 1 out]
      }
      event "cropY0": Value Change {
        n401 = event-data() -> ("NewVal"=w675:u64)  [unwired: 1 in, 5 out]
        n402 = local read "cropY1"() -> (w677:u64)
        n403 = Greater Or Equal?(x=w675, y=w677) -> (x >= y?=w676:bool)
        n404 = case shown="True" w676 {
          tunnel: w675 -> [_ w679]
          frame False {
          }
          frame True {
            n405 = Increment(x=w679) -> (x+1=w678:u64)
            n406 = local write "cropY1"(w678) -> ()
          }
        }
      }
      event "cropX1": Value Change {
        n407 = event-data() -> ("NewVal"=w680:u64)  [unwired: 1 in, 5 out]
        n408 = local read "cropX0"() -> (w682:u64)
        n409 = Less Or Equal?(x=w680, y=w682) -> (x <= y?=w681:bool)
        n410 = case shown="False" w681 {
          tunnel: w680 -> [_ w684]
          frame False {
          }
          frame True {
            n411 = Decrement(x=w684) -> (x-1=w683:u64)
            n412 = local write "cropX0"(w683) -> ()
          }
        }
      }
      event "cropY1": Value Change {
        n413 = event-data() -> ("NewVal"=w685:u64)  [unwired: 1 in, 5 out]
        n414 = local read "cropY0"() -> (w687:u64)
        n415 = Less Or Equal?(x=w685, y=w687) -> (x <= y?=w686:bool)
        n416 = case shown="True" w686 {
          tunnel: w685 -> [_ w689]
          frame False {
          }
          frame True {
            n417 = Decrement(x=w689) -> (x-1=w688:u64)
            n418 = local write "cropY0"(w688) -> ()
          }
        }
      }
    }
  }
